vi "lab1_readtxt.vi"() -> ()   [LabVIEW 2014]
panel:
  out "rx instant":string
  out "byte length":u32
  out "packet counter":u32
  out "found?":bool
  out "String":string
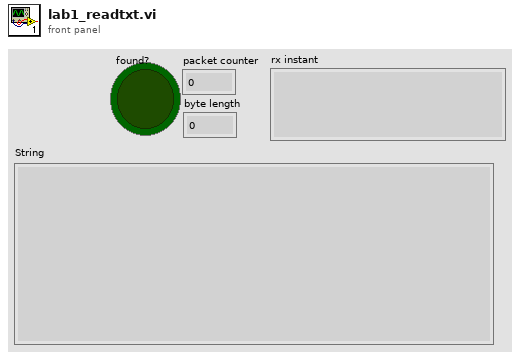
[diagram p1: front panel]
types:
  T1 = enum16{"open", "replace", "create", "open or create", "replace or create", "replace or create with confirmation"}
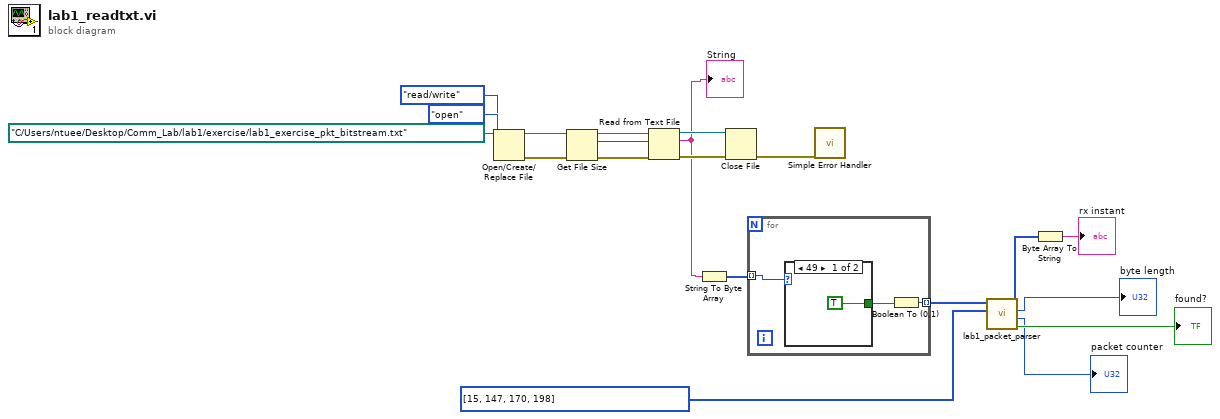
[diagram p0: block diagram]
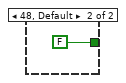
[diagram p2: hidden frame]
diagram:
  n1 = Open/Create/Replace File(file path (use dialog)=path "C:/Users/ntuee/Desktop/Comm_Lab/lab1/exercise/lab1_exercise_pkt_bitstream.txt", operation (0:open)=T1."open", access (0:read/write)=enum16{"read/write", "read-only", "write-only"}."read/write") -> (refnum out=w17:refnum<file>, error out=w16:errorcluster)  [unwired: 3 in, 1 out]
  n2 = Get File Size(file=w17, error in=w16) -> (refnum out=w13:refnum<file>, size (in bytes)=w14:i64, 0:w15:errorcluster)
  n3 = Read from Text File(file (use dialog)=w13, count=w14, error in=w15) -> (refnum out=w12:refnum<file>, text=w2:string, error out=w11:errorcluster)  [unwired: 1 in, 1 out]
  "String" <- w2
  n4 = String To Byte Array(string=w2) -> (unsigned byte array=w1:u8[])
  n5 = Close File(refnum=w12, error in=w11) -> (error out=w10:errorcluster)  [unwired: 1 out]
  n6 = for {
    tunnel: w1 -> [w23] mode=indexing
    tunnel: [w21] -> w9 mode=indexing
    n7 = case shown="49" w23 {
      tunnel: [TRUE FALSE] -> w22
      frame 49 {
      }
      frame 48, Default {
      }
    }
    n8 = Boolean To (0,1)(Boolean=w22) -> (0, 1=w21:i16)
  }
  n9 = call <vilib>:"Simple Error Handler.vi"("error in (no error)"=w10) -> ()  [unwired: 4 in, 5 out]
  n10 = call "lab1_packet_parser.vi"("preamble bytes"=u8[] [15, 147, 170, 198] ("Array"), "bitstream"=w9) -> ("Found?"=→"found?":bool, "packet counter"=→"packet counter":u32, "payload length(bytes)"=→"byte length":u32, "payload bytes"=w4:u8[])  [unwired: 6 in]
  n11 = Byte Array To String(unsigned byte array=w4) -> (string=→"rx instant":string)
